vi "Status to Boolean.vi"(4 "Status":string) -> (1 "Passed?":bool)   [LabVIEW 2015]
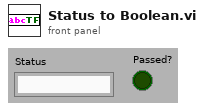
[diagram p1: front panel]
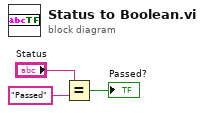
[diagram p0: block diagram]
diagram:
  n1 = Equal?(x="Status", y="Passed") -> (x = y?=→"Passed?":bool)
